vi "Sequence Add Column PDA.vi"(8 "error in (no error)":errorcluster, 11 "Connection Refnum":T1) -> (0 "error out":errorcluster, 3 "Connection Refnum":T1)   [LabVIEW 2011]
uses:
  SI.LIB/ODBC/SQL Controls/Connection Refnum.ctl
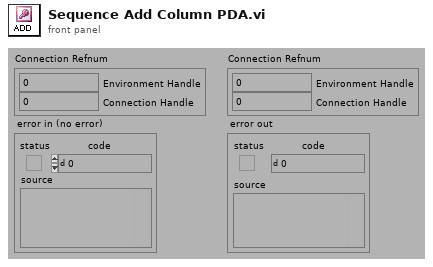
[diagram p1: front panel]
types:
  T1 = typedef "Connection Refnum.ctl" = cluster{"Environment Handle":i32, "Connection Handle":i32}
  T2 = typedef "Statement Refnum.ctl" = cluster{"Statement Handle":i32, "Parameter Number":u16}
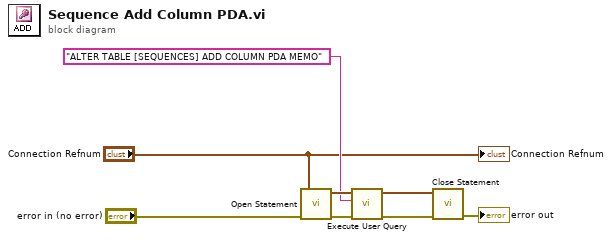
[diagram p0: block diagram]
diagram:
  n1 = call "Open Statement.vi"("error in (no error)"="error in (no error)", "Connection Refnum"="Connection Refnum") -> ("error out"=w7:errorcluster, "Statement Refnum"=w8:T2)  [unwired: 4 out]
  n2 = call "Execute User Query.vi"("error in (no error)"=w7, "User Query"="ALTER TABLE [SEQUENCES] ADD COLUMN PDA MEMO" ("format string"), "Statement Refnum"=w8) -> ("error out"=w5:errorcluster, "Statement Refnum"=w6:T2)  [unwired: 1 in, 2 out]
  n3 = call "Close Statement.vi"("error in (no error)"=w5, "Statement Refnum"=w6) -> ("error out"=→"error out":errorcluster)  [unwired: 5 out]
  "Connection Refnum" <- "Connection Refnum"
